vi "Get Tweets Search.vi"(8 "error in":errorcluster, 9 "Tweets to Read (10)":i32=10 min=0 max=200 step=1, 10 "Query":string, 11 "Twitter Handle In":T1={"OAuth Credentials"={"Consumer Key"="", "Signature Method"=enum."HMAC-SHA1", "Token"="", "Version"="", "Token Secret"="", "Consumer Secret"=""}, "since ID"="", "max ID"="", "Screen Name"=""}) -> (0 "error out":errorcluster, 1 "Actual Num of Tweets Read":i32, 2 "New Tweets Read":T4[](array[typedef]), 3 "Twitter Handle Out":T1={"OAuth Credentials"={"Consumer Key"="", "Signature Method"=enum."HMAC-SHA1", "Token"="", "Version"="", "Token Secret"="", "Consumer Secret"=""}, "since ID"="", "max ID"="", "Screen Name"=""}, 5 "Time Stamp of Newest Tweet":timestamp)   [LabVIEW 2011, in "i3-twitter.lvlib"]
uses:
  i3-twitter.lvlib
  Controls/Tweet.ctl
  Controls/Twitter Handle.ctl
  i3-oauth/Controls/OAuth Credentials.ctl
  i3-oauth/Controls/Signature Method.ctl
  i3-oauth/Controls/HTTP Method.ctl
  i3-json/JSON Parsing/Get Object Parameter Files/Get Object Parameter - Object.vi
  i3-json/JSON Parsing/Get Array Value at Index Files/Get Array Value at Index - Object.vi
  i3-json/JSON Parsing/Get Object Parameter Files/Get Object Parameter - String.vi
  i3-oauth/i3-oauth.lvlib
  <vilib>/httpClient/LabVIEWHTTPClient.lvlib
  i3-json/i3-json.lvlib
panel:
  out "Full URL":string
  out "body":string
  out "headers":string
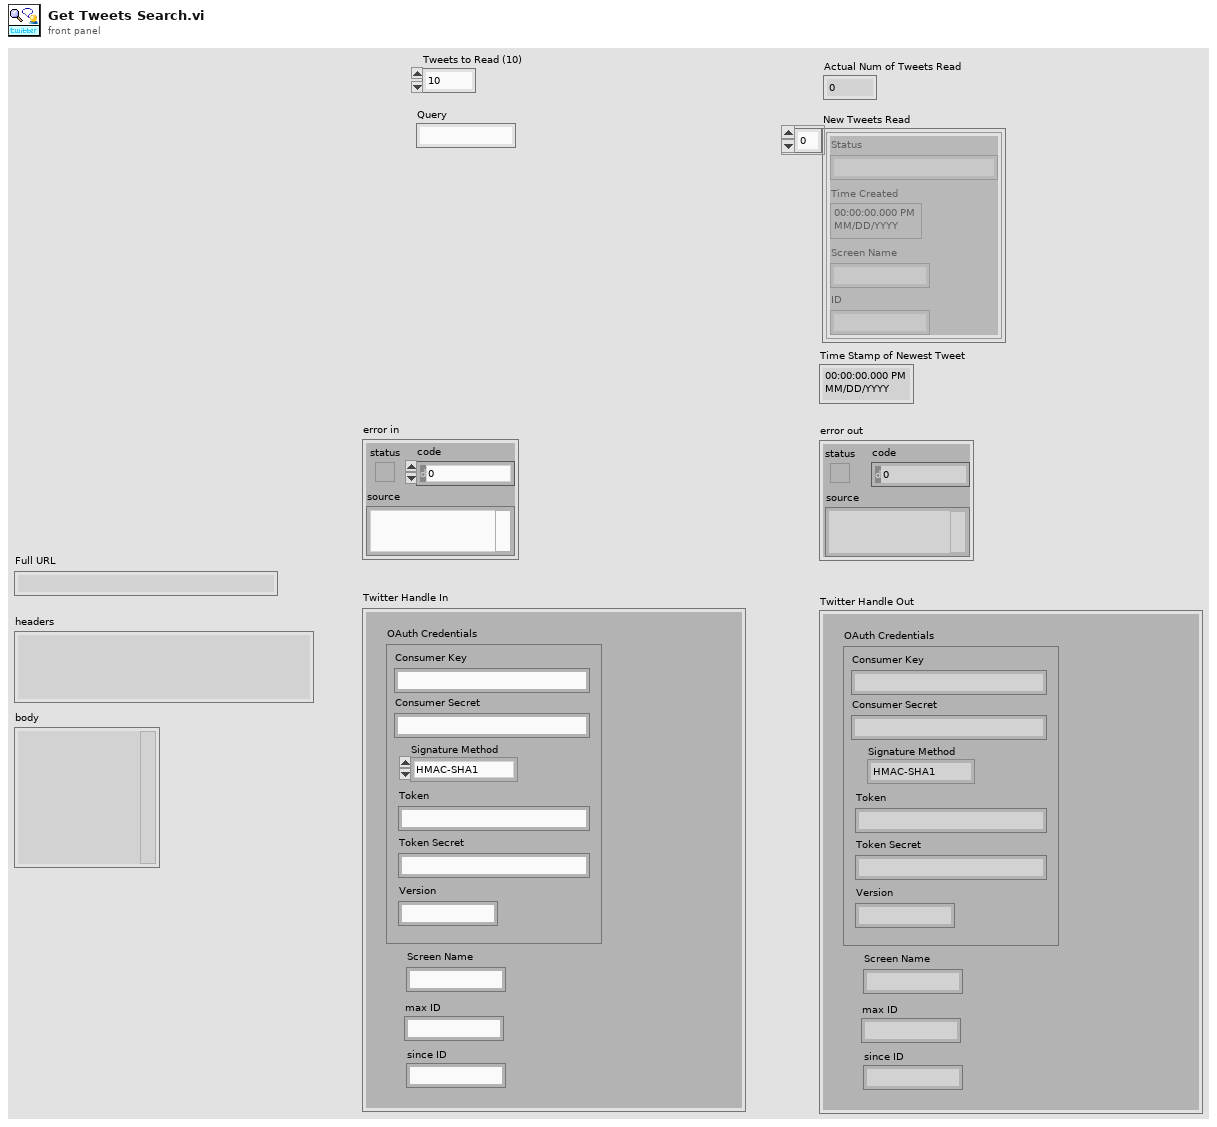
[diagram p1: front panel]
types:
  T1 = typedef "i3-twitter.lvlib/Twitter Handle.ctl" = cluster{"OAuth Credentials":T2, "since ID":string, "max ID":string, "Screen Name":string}
  T2 = typedef "i3-oauth.lvlib/OAuth Credentials.ctl" = cluster{"Consumer Key":string, "Signature Method":T3, "Token":string, "Version":string, "Token Secret":string, "Consumer Secret":string}
  T3 = typedef "i3-oauth.lvlib/Signature Method.ctl" = enum16{"HMAC-MD5", "HMAC-SHA1", "HMAC-SHA224", "HMAC-SHA256", "HMAC-SHA384", "HMAC-SHA512"}
  T4 = typedef "i3-twitter.lvlib/Tweet.ctl" = cluster{"Status":string, "Time Created":timestamp, "Screen Name":string, "ID":string}
  T5 = typedef "i3-oauth.lvlib/HTTP Method.ctl" = enum16{"GET", "POST", "PUT", "DELETE"}
  T6 = typedef "i3-oauth.lvlib/key-value-pairs.ctl" = cluster{"key":string, "value":string}
  T7 = typedef "LabVIEWHTTPClient.lvlib/ClientHandle.ctl" = refnum<k1>
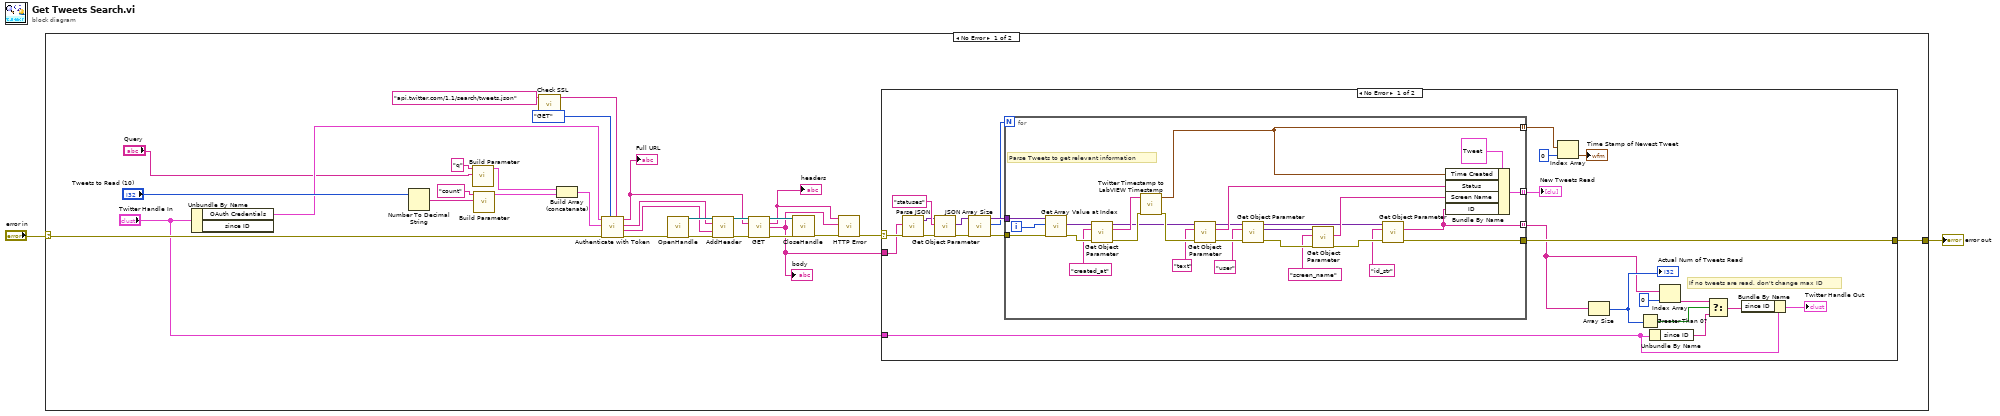
[diagram p0: block diagram]
diagram:
  n1 = case shown="No Error" "error in" {
    selector: "error in" -> [w31 w84]
    tunnel: [w13 w84] -> w2
    frame No Error {
      n2 = Unbundle By Name("Twitter Handle In") -> ("OAuth Credentials"=w10:T2)  [unwired: 1 out]
      n3 = Number To Decimal String(number="Tweets to Read (10)") -> (decimal integer string=w19:string)  [unwired: 1 in]
      n4 = call "Build Parameter.vi"("Value"="Query", "Key"="q") -> ("Parameter Array"=w4:T6[])  [unwired: 9 in]
      n5 = call "Build Parameter.vi"("Value"=w19, "Key"="count") -> ("Parameter Array"=w7:T6[])  [unwired: 9 in]
      n6 = call "Check SSL.vi"("Input URL"="api.twitter.com/1.1/search/tweets.json" ("Base URL")) -> ("Output URL"=w8:string)  [unwired: 8 in]
      n7 = Build Array (concatenate)(w4, w7) -> (w18:T6[])
      n8 = call "Authenticate with Token.vi"("Base URL"=w8, "HTTP Method"=HTTP_Method."GET", "error in (no error)"=w31, "URL Parameters"=w18, "OAuth Credentials"=w10) -> ("error out"=w17:errorcluster, "Header Value"=w23:string, "Header Parameter"=w24:string, "Full URL"=w22:string)  [unwired: 2 in, 1 out]
      "Full URL" <- w22
      n9 = call <vilib>:"OpenHandle.vi"("error in (no error)"=w17) -> ("client handle out"=w30:T7, "error out"=w29:errorcluster)  [unwired: 13 in]
      n10 = call <vilib>:"AddHeader.vi"("client handle"=w30, "header"=w24, "value"=w23, "error in (no error)"=w29) -> ("client handle out"=w28:T7, "error out"=w27:errorcluster)  [unwired: 10 in]
      n11 = call <vilib>:"GET.vi"("client handle"=w28, "url"=w22, "error in (no error)"=w27) -> ("client handle out"=w26:T7, "headers"=w16:string, "body"=w12:string, "error out"=w25:errorcluster)  [unwired: 9 in]
      "body" <- w12
      "headers" <- w16
      n12 = call <vilib>:"CloseHandle.vi"("client handle"=w26, "error in (no error)"=w25) -> ("error out"=w15:errorcluster)  [unwired: 13 in]
      n13 = call "HTTP Error.vi"("error in (no error)"=w15, "Body"=w12, "Header"=w16) -> ("error out"=w14:errorcluster)  [unwired: 6 in, 2 out]
      n14 = case shown="No Error" w14 {
        selector: w14 -> [w51 w83]
        tunnel: [w50 w83] -> w13
        tunnel: w12 -> [w49 _]
        tunnel: "Twitter Handle In" -> [w32 _]
        frame No Error {
          # "If no tweets are read, don't change max ID"
          n15 = call "Parse JSON.vi"("error in (no error)"=w51, "JSON String"=w49) -> ("error out"=w41:errorcluster, "JSON Tree"=w42:variant)  [unwired: 6 in, 2 out]
          n16 = call-poly "Get Object Parameter.vi"("error in (no error)"=w41, "Parameter Name"="statuses", "JSON Tree In (JSON Object)"=w42) -> ("error out"=w45:errorcluster, "JSON Object"=w44:variant)  [unwired: 5 in, 2 out]
          n17 = call "JSON Array Size.vi"("error in (no error)"=w45, "JSON Tree In (JSON Array)"=w44) -> ("error out"=w53:errorcluster, "Array Size"=w54:i32, "JSON Tree Passthrough (JSON Array)"=w55:variant)  [unwired: 7 in]
          n18 = for {
            N: w54 -> [_]
            tunnel: w53 -> [w66]
            tunnel: [w69] -> w52 mode=indexing
            tunnel: [w68] -> w50
            tunnel: w55 -> [w65]
            tunnel: [w64] -> w48 mode=indexing
            tunnel: [w56] -> w33 mode=indexing
            i -> [w71]
            # "Parse Tweets to get relevant information"
            n19 = call-poly "Get Array Value at Index.vi"("error in (no error)"=w66, "Index"=w71, "JSON Tree In (JSON Array)"=w65) -> ("error out"=w78:errorcluster, "JSON Object"=w62:variant)  [unwired: 5 in, 2 out]
            n20 = call-poly "Get Object Parameter.vi"("error in (no error)"=w78, "Parameter Name"="created_at", "JSON Tree In (JSON Object)"=w62) -> ("error out"=w61:errorcluster, "String Value"=w60:string, "JSON Tree Out Passthrough"=w59:variant)  [unwired: 5 in, 1 out]
            n21 = call "Twitter Timestamp to LabVIEW Timestamp.vi"("error in"=w61, "Twitter Time Stamp"=w60) -> ("error out"=w79:errorcluster, "LabVIEW Time Stamp"=w64:timestamp)  [unwired: 6 in]
            n22 = call-poly "Get Object Parameter.vi"("error in (no error)"=w79, "Parameter Name"="text", "JSON Tree In (JSON Object)"=w59) -> ("error out"=w80:errorcluster, "String Value"=w67:string, "JSON Tree Out Passthrough"=w58:variant)  [unwired: 5 in, 1 out]
            n23 = call-poly "Get Object Parameter.vi"("error in (no error)"=w80, "Parameter Name"="user", "JSON Tree In (JSON Object)"=w58) -> ("error out"=w81:errorcluster, "JSON Object"=w63:variant, "JSON Tree Out Passthrough"=w57:variant)  [unwired: 5 in, 1 out]
            n24 = call-poly "Get Object Parameter.vi"("error in (no error)"=w81, "Parameter Name"="screen_name", "JSON Tree In (JSON Object)"=w63) -> ("error out"=w82:errorcluster, "String Value"=w74:string)  [unwired: 5 in, 2 out]
            n25 = call-poly "Get Object Parameter.vi"("error in (no error)"=w82, "Parameter Name"="id_str", "JSON Tree In (JSON Object)"=w57) -> ("error out"=w68:errorcluster, "String Value"=w56:string)  [unwired: 5 in, 2 out]
            n26 = Bundle By Name(cluster=T4 {"Status"="", "Time Created"=timestamp(0 s since 1904-01-01), "Screen Name"="", "ID"=""}, "Time Created"=w64, "Status"=w67, "Screen Name"=w74, "ID"=w56) -> (w69:T4)
          }
          "New Tweets Read" <- w52
          n27 = Index Array(array=w48, index=0) -> (element=→"Time Stamp of Newest Tweet":timestamp)
          n28 = Array Size(array=w33) -> (size(s)=w39:i32)
          "Actual Num of Tweets Read" <- w39
          n29 = Greater Than 0?(x=w39) -> (x > 0?=w40:bool)
          n30 = Unbundle By Name(w32) -> ("since ID"=w34:string)
          n31 = Index Array(array=w33, index=0) -> (element=w38:string)
          n32 = Select(t=w38, s=w40, f=w34) -> (s? t:f=w37:string)
          n33 = Bundle By Name(cluster=w32, "since ID"=w37) -> (→"Twitter Handle Out":T1)
        }
        frame Error {
        }
      }
    }
    frame Error {
    }
  }
  "error out" <- w2
